vi "CCD Basic 1 Shot.vi"() -> ()   [LabVIEW 2020]
panel:
  out "ts [0] read":errorcluster
  out "st [0]  err":errorcluster
  in  "Exposuretime (s)":dbl=0.5 format="%.2f"
  out "PixelOverflow":bool
  out "InitialArray Length":i32=16384
  out "ld":i32=16
  out "sd":i32=1024
  out "Array Length":i32=1024
  out "?":i32[](graph)=[1198, 1190, 1193, 1194, 1189, 1188, 1196, 1190, 1202, 1191, 1193, 1192, 1199, 1189, 1194, 1189, 1197, 1191, 1187, 1192, 1195, 1189, 1195, 1191, 1199, 1194, 1192, 1191, 1193, 1197, 1193, 1193, 1194, 1200, 1191, 1190, 1187, 1195, 1189, 1188, 1191, 1194, 1187, 1192, 1198, 1193, 1190, 1192, 1190, 1193, 1191, 1190, 1191, 1189, 1192, 1194, 1190, 1193, 1193, 1191, 1194, 1182, 1190, 1188, 1199, 1192, 1196, 1195, 1186, 1189, 1188, 1185, 1194, 1187, 1193, 1194, 1190, 1189, 1189, 1187, 1196, 1195, 1191, 1197, 1192, 1200, 1187, 1194, 1189, 1193, 1195, 1196, 1186, 1192, 1190, 1194, 1194, 1190, 1191, 1193, 1197, 1197, 1185, 1199, 1190, 1195, 1196, 1184, 1193, 1193, 1193, 1191, 1189, 1190, 1199, 1193, 1191, 1194, 1191, 1192, 1186, 1190, 1194, 1189, 1194, 1190, 1191, 1192, 1192, 1196, 1192, 1192, 1189, 1193, 1198, 1186, 1191, 1193, 1187, 1194, 1190, 1190, 1191, 1189, 1194, 1195, 1189, 1192, 1185, 1193, 1192, 1192, 1189, 1191, 1191, 1190, 1196, 1194, 1193, 1191, 1189, 1191, 1196, 1192, 1192, 1189, 1196, 1191, 1193, 1192, 1188, 1190, 1194, 1192, 1185, 1191, 1194, 1191, 1189, 1195, 1192, 1196, 1190, 1193, 1191, 1189, 1194, 1195, 1191, 1187, 1190, 1196, 1196, 1192, 1197, 1191, 1189, 1192, 1192, 1200, 1192, 1193, 1190, 1192, 1187, 1198, 1186, 1196, 1201, 1199, 1200, 1191, 1196, 1200, 1192, 1191, 1193, 1185, 1192, 1194, 1186, 1190, 1188, 1189, 1201, 1197, 1191, 1194, 1193, 1194, 1195, 1198, 1200, 1192, 1192, 1193, 1193, 1195, 1187, 1193, 1192, 1187, 1189, 1186, 1191, 1197, 1191, 1200, 1194, 1192, 1187, 1196, 1191, 1191, 1196, 1187, 1190, 1193, 1189, 1193, 1190, 1188, 1188, 1190, 1197, 1188, 1191, 1195, 1188, 1191, 1188, 1194, 1193, 1187, 1200, 1192, 1197, 1190, 1196, 1200, 1191, 1189, 1193, 1189, 1186, 1196, 1185, 1198, 1195, 1186, 1191, 1197, 1191, 1193, 1195, 1193, 1191, 1198, 1189, 1183, 1200, 1197, 1192, 1192, 1192, 1196, 1191, 1190, 1194, 1188, 1198, 1193, 1195, 1190, 1187, 1192, 1191, 1195, 1188, 1190, 1191, 1187, 1189, 1185, 1189, 1196, 1198, 1191, 1190, 1196, 1197, 1193, 1187, 1186, 1195, 1191, 1193, 1192, 1196, 1190, 1192, 1192, 1192, 1190, 1195, 1192, 1191, 1193, 1197, 1184, 1190, 1188, 1192, 1194, 1190, 1193, 1195, 1195, 1194, 1189, 1193, 1191, 1194, 1186, 1189, 1192, 1191, 1182, 1190, 1197, 1194, 1188, 1193, 1191, 1186, 1194, 1197, 1193, 1191, 1187, 1194, 1194, 1191, 1189, 1195, 1194, 1189, 1196, 1187, 1186, 1192, 1194, 1196, 1191, 1193, 1191, 1188, 1190, 1199, 1198, 1196, 1196, 1190, 1194, 1191, 1194, 1187, 1195, 1190, 1194, 1196, 1194, 1189, 1193, 1189, 1194, 1189, 1195, 1192, 1194, 1193, 1191, 1197, 1187, 1189, 1189, 1188, 1197, 1192, 1189, 1193, 1194, 1183, 1202, 1187, 1192, 1184, 1188, 1186, 1193, 1189, 1195, 1189, 1193, 1197, 1189, 1194, 1191, 1194, 1192, 1191, 1191, 1196, 1194, 1190, 1193, 1192, 1195, 1197, 1198, 1193, 1202, 1196, 1194, 1194, 1190, 1193, 1190, 1195, 1192, 1187, 1194, 1197, 1190, 1194, 1189, 1198, 1192, 1191, 1192, 1192, 1191, 1191, 1193, 1191, 1191, 1198, 1186, 1192, 1185, 1185, 1188, 1194, 1196, 1194, 1195, 1190, 1194, 1191, 1190, 1195, 1191, 1191, 1195, 1192, 1194, 1201, 1187, 1191, 1195, 1187, 1192, 1192, 1193, 1200, 1188, 1189, 1189, 1197, 1189, 1188, 1197, 1195, 1191, 1189, 1190, 1195, 1189, 1191, 1194, 1186, 1192, 1190, 1191, 1188, 1195, 1192, 1191, 1191, 1199, 1190, 1190, 1190, 1192, 1187, 1193, 1197, 1197, 1186, 1193, 1189, 1192, 1197, 1184, 1187, 1188, 1192, 1192, 1192, 1189, 1192, 1190, 1194, 1191, 1186, 1196, 1194, 1189, 1193, 1191, 1186, 1189, 1193, 1195, 1196, 1197, 1199, 1194, 1190, 1193, 1194, 1190, 1198, 1196, 1194, 1195, 1194, 1184, 1188, 1195, 1197, 1190, 1194, 1190, 1191, 1195, 1198, 1188, 1193, 1194, 1195, 1198, 1195, 1191, 1197, 1192, 1198, 1190, 1196, 1191, 1194, 1188, 1189, 1198, 1192, 1198, 1195, 1185, 1191, 1193, 1192, 1197, 1195, 1195, 1195, 1193, 1190, 1190, 1190, 1198, 1195, 1191, 1194, 1190, 1190, 1194, 1194, 1195, 1192, 1190, 1194, 1195, 1192, 1192, 1194, 1189, 1192, 1193, 1188, 1194, 1195, 1196, 1193, 1192, 1201, 1191, 1198, 1197, 1191, 1192, 1191, 1194, 1193, 1188, 1192, 1189, 1183, 1189, 1190, 1192, 1189, 1196, 1193, 1197, 1185, 1193, 1189, 1191, 1196, 1195, 1193, 1193, 1191, 1189, 1193, 1192, 1192, 1192, 1190, 1191, 1193, 1193, 1197, 1195, 1189, 1193, 1188, 1194, 1197, 1194, 1195, 1196, 1190, 1194, 1188, 1197, 1195, 1191, 1195, 1192, 1194, 1188, 1190, 1197, 1197, 1191, 1187, 1197, 1191, 1193, 1188, 1191, 1194, 1193, 1195, 1192, 1195, 1189, 1193, 1193, 1195, 1190, 1192, 1196, 1188, 1187, 1193, 1192, 1192, 1194, 1185, 1199, 1190, 1193, 1191, 1198, 1189, 1190, 1191, 1190, 1193, 1195, 1186, 1190, 1193, 1191, 1189, 1197, 1193, 1198, 1190, 1192, 1193, 1191, 1196, 1193, 1196, 1190, 1190, 1198, 1192, 1199, 1198, 1190, 1191, 1191, 1196, 1190, 1196, 1195, 1191, 1196, 1195, 1193, 1190, 1190, 1195, 1193, 1187, 1197, 1185, 1191, 1189, 1191, 1193, 1192, 1188, 1196, 1193, 1191, 1193, 1193, 1190, 1192, 1192, 1192, 1195, 1191, 1195, 1189, 1189, 1191, 1191, 1185, 1192, 1191, 1193, 1201, 1199, 1197, 1206, 1201, 1207, 1200, 1198, 1195, 1188, 1194, 1186, 1190, 1197, 1188, 1193, 1196, 1193, 1192, 1192, 1188, 1196, 1186, 1193, 1194, 1188, 1190, 1190, 1192, 1190, 1191, 1191, 1200, 1192, 1199, 1193, 1190, 1190, 1199, 1187, 1193, 1190, 1188, 1194, 1194, 1196, 1194, 1195, 1190, 1187, 1187, 1196, 1193, 1199, 1190, 1193, 1193, 1191, 1198, 1192, 1193, 1192, 1193, 1189, 1189, 1197, 1189, 1194, 1193, 1192, 1185, 1198, 1193, 1189, 1192, 1193, 1196, 1190, 1195, 1189, 1196, 1198, 1190, 1191, 1193, 1186, 1189, 1195, 1188, 1197, 1188, 1191, 1185, 1190, 1193, 1188, 1198, 1192, 1193, 1194, 1194, 1189, 1184, 1193, 1199, 1193, 1192, 1193, 1190, 1196, 1191, 1192, 1189, 1194, 1188, 1189, 1190, 1190, 1192, 1195, 1188, 1190, 1192, 1189, 1197, 1192, 1194, 1187, 1196, 1192, 1194, 1185, 1187, 1187, 1191, 1195, 1190, 1186, 1183, 1194, 1194, 1192, 1192, 1188, 1193, 1195, 1189, 1190, 1191, 1192, 1196, 1186, 1195, 1191, 1185, 1191, 1187, 1190, 1188, 1189, 1187, 1196, 1191, 1190, 1191, 1190, 1196, 1195, 1186, 1187, 1187, 1188, 1194, 1192, 1192, 1192, 1189, 1192, 1191, 1188, 1188, 1187, 1187, 1190, 1186, 1191, 1195, 1192, 1196, 1193, 1192, 1191, 1189, 1187, 1193, 1188, 1189, 1194, 1191, 1185, 1193, 1191, 1196, 1196, 1199, 1195, 1211]
  in  "Setup String":string="ldu,0,256,16;sdu,0,1024,1024;cl0;omrm;sron"
  out "The Data":i32[](array[numeric])=[1198, 1190, 1193, 1194, 1189, 1188, 1196, 1190, 1202, 1191, 1193, 1192, 1199, 1189, 1194, 1189, 1197, 1191, 1187, 1192, 1195, 1189, 1195, 1191, 1199, 1194, 1192, 1191, 1193, 1197, 1193, 1193, 1194, 1200, 1191, 1190, 1187, 1195, 1189, 1188, 1191, 1194, 1187, 1192, 1198, 1193, 1190, 1192, 1190, 1193, 1191, 1190, 1191, 1189, 1192, 1194, 1190, 1193, 1193, 1191, 1194, 1182, 1190, 1188, 1199, 1192, 1196, 1195, 1186, 1189, 1188, 1185, 1194, 1187, 1193, 1194, 1190, 1189, 1189, 1187, 1196, 1195, 1191, 1197, 1192, 1200, 1187, 1194, 1189, 1193, 1195, 1196, 1186, 1192, 1190, 1194, 1194, 1190, 1191, 1193, 1197, 1197, 1185, 1199, 1190, 1195, 1196, 1184, 1193, 1193, 1193, 1191, 1189, 1190, 1199, 1193, 1191, 1194, 1191, 1192, 1186, 1190, 1194, 1189, 1194, 1190, 1191, 1192, 1192, 1196, 1192, 1192, 1189, 1193, 1198, 1186, 1191, 1193, 1187, 1194, 1190, 1190, 1191, 1189, 1194, 1195, 1189, 1192, 1185, 1193, 1192, 1192, 1189, 1191, 1191, 1190, 1196, 1194, 1193, 1191, 1189, 1191, 1196, 1192, 1192, 1189, 1196, 1191, 1193, 1192, 1188, 1190, 1194, 1192, 1185, 1191, 1194, 1191, 1189, 1195, 1192, 1196, 1190, 1193, 1191, 1189, 1194, 1195, 1191, 1187, 1190, 1196, 1196, 1192, 1197, 1191, 1189, 1192, 1192, 1200, 1192, 1193, 1190, 1192, 1187, 1198, 1186, 1196, 1201, 1199, 1200, 1191, 1196, 1200, 1192, 1191, 1193, 1185, 1192, 1194, 1186, 1190, 1188, 1189, 1201, 1197, 1191, 1194, 1193, 1194, 1195, 1198, 1200, 1192, 1192, 1193, 1193, 1195, 1187, 1193, 1192, 1187, 1189, 1186, 1191, 1197, 1191, 1200, 1194, 1192, 1187, 1196, 1191, 1191, 1196, 1187, 1190, 1193, 1189, 1193, 1190, 1188, 1188, 1190, 1197, 1188, 1191, 1195, 1188, 1191, 1188, 1194, 1193, 1187, 1200, 1192, 1197, 1190, 1196, 1200, 1191, 1189, 1193, 1189, 1186, 1196, 1185, 1198, 1195, 1186, 1191, 1197, 1191, 1193, 1195, 1193, 1191, 1198, 1189, 1183, 1200, 1197, 1192, 1192, 1192, 1196, 1191, 1190, 1194, 1188, 1198, 1193, 1195, 1190, 1187, 1192, 1191, 1195, 1188, 1190, 1191, 1187, 1189, 1185, 1189, 1196, 1198, 1191, 1190, 1196, 1197, 1193, 1187, 1186, 1195, 1191, 1193, 1192, 1196, 1190, 1192, 1192, 1192, 1190, 1195, 1192, 1191, 1193, 1197, 1184, 1190, 1188, 1192, 1194, 1190, 1193, 1195, 1195, 1194, 1189, 1193, 1191, 1194, 1186, 1189, 1192, 1191, 1182, 1190, 1197, 1194, 1188, 1193, 1191, 1186, 1194, 1197, 1193, 1191, 1187, 1194, 1194, 1191, 1189, 1195, 1194, 1189, 1196, 1187, 1186, 1192, 1194, 1196, 1191, 1193, 1191, 1188, 1190, 1199, 1198, 1196, 1196, 1190, 1194, 1191, 1194, 1187, 1195, 1190, 1194, 1196, 1194, 1189, 1193, 1189, 1194, 1189, 1195, 1192, 1194, 1193, 1191, 1197, 1187, 1189, 1189, 1188, 1197, 1192, 1189, 1193, 1194, 1183, 1202, 1187, 1192, 1184, 1188, 1186, 1193, 1189, 1195, 1189, 1193, 1197, 1189, 1194, 1191, 1194, 1192, 1191, 1191, 1196, 1194, 1190, 1193, 1192, 1195, 1197, 1198, 1193, 1202, 1196, 1194, 1194, 1190, 1193, 1190, 1195, 1192, 1187, 1194, 1197, 1190, 1194, 1189, 1198, 1192, 1191, 1192, 1192, 1191, 1191, 1193, 1191, 1191, 1198, 1186, 1192, 1185, 1185, 1188, 1194, 1196, 1194, 1195, 1190, 1194, 1191, 1190, 1195, 1191, 1191, 1195, 1192, 1194, 1201, 1187, 1191, 1195, 1187, 1192, 1192, 1193, 1200, 1188, 1189, 1189, 1197, 1189, 1188, 1197, 1195, 1191, 1189, 1190, 1195, 1189, 1191, 1194, 1186, 1192, 1190, 1191, 1188, 1195, 1192, 1191, 1191, 1199, 1190, 1190, 1190, 1192, 1187, 1193, 1197, 1197, 1186, 1193, 1189, 1192, 1197, 1184, 1187, 1188, 1192, 1192, 1192, 1189, 1192, 1190, 1194, 1191, 1186, 1196, 1194, 1189, 1193, 1191, 1186, 1189, 1193, 1195, 1196, 1197, 1199, 1194, 1190, 1193, 1194, 1190, 1198, 1196, 1194, 1195, 1194, 1184, 1188, 1195, 1197, 1190, 1194, 1190, 1191, 1195, 1198, 1188, 1193, 1194, 1195, 1198, 1195, 1191, 1197, 1192, 1198, 1190, 1196, 1191, 1194, 1188, 1189, 1198, 1192, 1198, 1195, 1185, 1191, 1193, 1192, 1197, 1195, 1195, 1195, 1193, 1190, 1190, 1190, 1198, 1195, 1191, 1194, 1190, 1190, 1194, 1194, 1195, 1192, 1190, 1194, 1195, 1192, 1192, 1194, 1189, 1192, 1193, 1188, 1194, 1195, 1196, 1193, 1192, 1201, 1191, 1198, 1197, 1191, 1192, 1191, 1194, 1193, 1188, 1192, 1189, 1183, 1189, 1190, 1192, 1189, 1196, 1193, 1197, 1185, 1193, 1189, 1191, 1196, 1195, 1193, 1193, 1191, 1189, 1193, 1192, 1192, 1192, 1190, 1191, 1193, 1193, 1197, 1195, 1189, 1193, 1188, 1194, 1197, 1194, 1195, 1196, 1190, 1194, 1188, 1197, 1195, 1191, 1195, 1192, 1194, 1188, 1190, 1197, 1197, 1191, 1187, 1197, 1191, 1193, 1188, 1191, 1194, 1193, 1195, 1192, 1195, 1189, 1193, 1193, 1195, 1190, 1192, 1196, 1188, 1187, 1193, 1192, 1192, 1194, 1185, 1199, 1190, 1193, 1191, 1198, 1189, 1190, 1191, 1190, 1193, 1195, 1186, 1190, 1193, 1191, 1189, 1197, 1193, 1198, 1190, 1192, 1193, 1191, 1196, 1193, 1196, 1190, 1190, 1198, 1192, 1199, 1198, 1190, 1191, 1191, 1196, 1190, 1196, 1195, 1191, 1196, 1195, 1193, 1190, 1190, 1195, 1193, 1187, 1197, 1185, 1191, 1189, 1191, 1193, 1192, 1188, 1196, 1193, 1191, 1193, 1193, 1190, 1192, 1192, 1192, 1195, 1191, 1195, 1189, 1189, 1191, 1191, 1185, 1192, 1191, 1193, 1201, 1199, 1197, 1206, 1201, 1207, 1200, 1198, 1195, 1188, 1194, 1186, 1190, 1197, 1188, 1193, 1196, 1193, 1192, 1192, 1188, 1196, 1186, 1193, 1194, 1188, 1190, 1190, 1192, 1190, 1191, 1191, 1200, 1192, 1199, 1193, 1190, 1190, 1199, 1187, 1193, 1190, 1188, 1194, 1194, 1196, 1194, 1195, 1190, 1187, 1187, 1196, 1193, 1199, 1190, 1193, 1193, 1191, 1198, 1192, 1193, 1192, 1193, 1189, 1189, 1197, 1189, 1194, 1193, 1192, 1185, 1198, 1193, 1189, 1192, 1193, 1196, 1190, 1195, 1189, 1196, 1198, 1190, 1191, 1193, 1186, 1189, 1195, 1188, 1197, 1188, 1191, 1185, 1190, 1193, 1188, 1198, 1192, 1193, 1194, 1194, 1189, 1184, 1193, 1199, 1193, 1192, 1193, 1190, 1196, 1191, 1192, 1189, 1194, 1188, 1189, 1190, 1190, 1192, 1195, 1188, 1190, 1192, 1189, 1197, 1192, 1194, 1187, 1196, 1192, 1194, 1185, 1187, 1187, 1191, 1195, 1190, 1186, 1183, 1194, 1194, 1192, 1192, 1188, 1193, 1195, 1189, 1190, 1191, 1192, 1196, 1186, 1195, 1191, 1185, 1191, 1187, 1190, 1188, 1189, 1187, 1196, 1191, 1190, 1191, 1190, 1196, 1195, 1186, 1187, 1187, 1188, 1194, 1192, 1192, 1192, 1189, 1192, 1191, 1188, 1188, 1187, 1187, 1190, 1186, 1191, 1195, 1192, 1196, 1193, 1192, 1191, 1189, 1187, 1193, 1188, 1189, 1194, 1191, 1185, 1193, 1191, 1196, 1196, 1199, 1195, 1211]
  in  "CCD GPIB Address":refnum<visa-resource-name>
  # "Note: Check Summing of Data!"
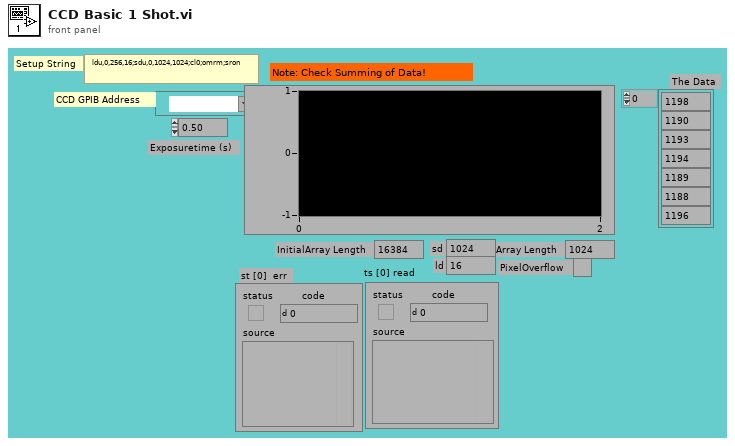
[diagram p1: front panel]
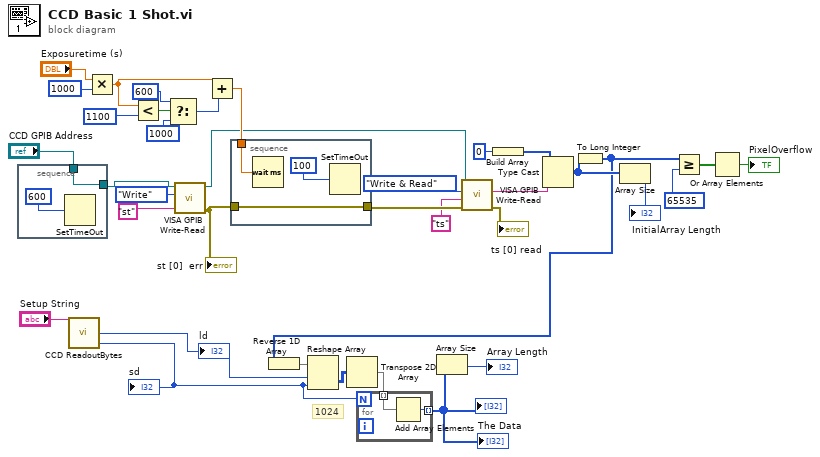
[diagram p0: block diagram]
diagram:
  # "1024"
  n1 = stacked-sequence {
    tunnel: [w37] -> w3
    tunnel: "CCD GPIB Address" -> [w37]
    frame #0 {
      n2 = SetTimeOut(1:600) -> ()  [unwired: 1 out]
    }
  }
  n3 = call "CCD ReadoutBytes.vi"("CCD Setup String"="Setup String") -> ("LD Bytes"=w8:i32, "SD Bytes"=w7:i32)  [unwired: 1 in, 2 out]
  "sd" <- w7
  "ld" <- w8
  n4 = Multiply(x="Exposuretime (s)", y=1000) -> (x*y=w29:dbl)
  n5 = Less?(x=w29, y=1100) -> (x < y?=w31:bool)
  n6 = Select(t=u32 600, s=w31, f=u32 1000 ("Added are a minimum of 600ms")) -> (s? t:f=w28:u32)
  n7 = call "VISA GPIB Write-Read.vi"("Command"="st", "Action"=enum16{"Write", "Read", "Write & Read"}."Write", "VISA resource name"=w3) -> ("error out"=w26:errorcluster, "dup VISA Session"=w1:refnum<visa-resource-name>)  [unwired: 5 in, 2 out]
  "st [0]  err" <- w26
  n8 = Add(x=w29, y=w28) -> (x+y=w27:dbl)
  n9 = stacked-sequence {
    tunnel: w27 -> [w41]
    tunnel: w26 -> [w40]
    tunnel: [w40] -> w24
    frame #0 {
      n10 = Wait (ms)(milliseconds to wait=w41) -> ()  [unwired: 1 out]
      n11 = SetTimeOut(1:100) -> ()  [unwired: 1 out]
    }
  }
  n12 = call "VISA GPIB Write-Read.vi"("error in (no error)"=w24, "Command"="ts" ("String to Write"), "Action"=enum16{"Write", "Read", "Write & Read"}."Write & Read", "VISA resource name"=w1) -> ("error out"=→"ts [0] read":errorcluster, "String Returned"=w17:string)  [unwired: 4 in, 2 out]
  n13 = Build Array(u16 0) -> (w18:u16[])
  n14 = Type Cast(type=w18, x=w17) -> (*(type *) &x=w20:u16[])
  n15 = To Long Integer(number=w20) -> (32bit integer=w9:i32[])
  n16 = Reverse 1D Array(array=w9) -> (reversed array=w10:i32[])
  n17 = Reshape Array(w10, w8, w7) -> (w11:i32[][])
  n18 = Transpose 2D Array(2D array=w11) -> (transposed array=w12:i32[][])
  n19 = for {
    N: w7 -> [_]
    tunnel: w12 -> [w43] mode=indexing
    tunnel: [w42] -> w6 mode=indexing
    n20 = Add Array Elements(numeric array=w43) -> (sum=w42:i32)
  }
  "The Data" <- w6
  "?" <- w6
  n21 = Array Size(array=w6) -> (size(s)=→"Array Length":i32)
  n22 = Array Size(array=w20) -> (size(s)=→"InitialArray Length":i32)
  n23 = Greater Or Equal?(x=w9, y=65535) -> (x >= y?=w14:bool[])
  n24 = Or Array Elements(Boolean array=w14) -> (logical OR=→"PixelOverflow":bool)
